vi "ESA-C Get Absolute Velocity.vi"(1 "Axis":i32, 2 "Velocity (V)":dbl) -> (0 "Velocity (µm)":dbl)   [LabVIEW 2010]
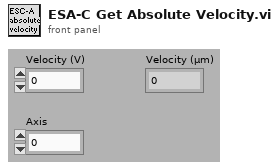
[diagram p1: front panel]
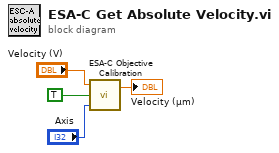
[diagram p0: block diagram]
diagram:
  n1 = call "ESA-C Objective Calibration.vi"("Axis"="Axis", "Is Voltage?"=TRUE, "Input Value"="Velocity (V)") -> ("Output Value"=→"Velocity (µm)":dbl)  [unwired: 1 in]
